vi "TestData_FileFormatCheck.vi"(8 "错误输入":errorcluster, 10 "Format Err":path, 11 "File":path) -> (0 "错误输出":errorcluster, 1 "Err_Count":i32, 3 "OK_Data":string[](array[string]))   [LabVIEW 2012, in "Lib_UEL.ATE.lvlib" / "Lib_TestData.lvlib"]
uses:
  Lib_TestData.lvlib
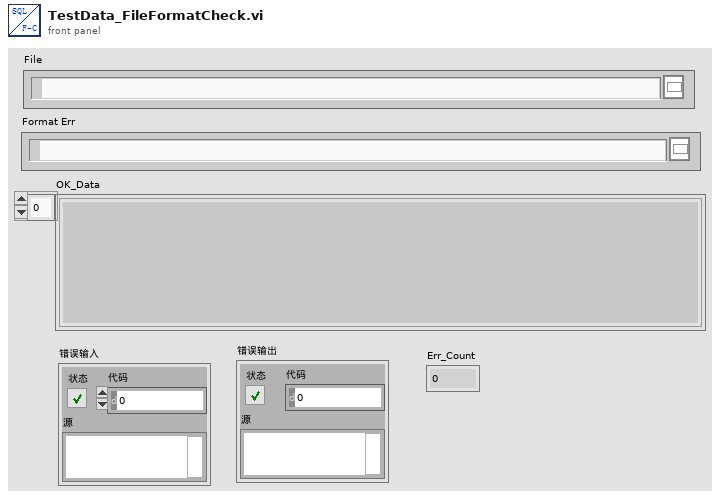
[diagram p1: front panel]
types:
  T1 = enum16{"open", "replace", "create", "open or create", "replace or create", "replace or create with confirmation"}
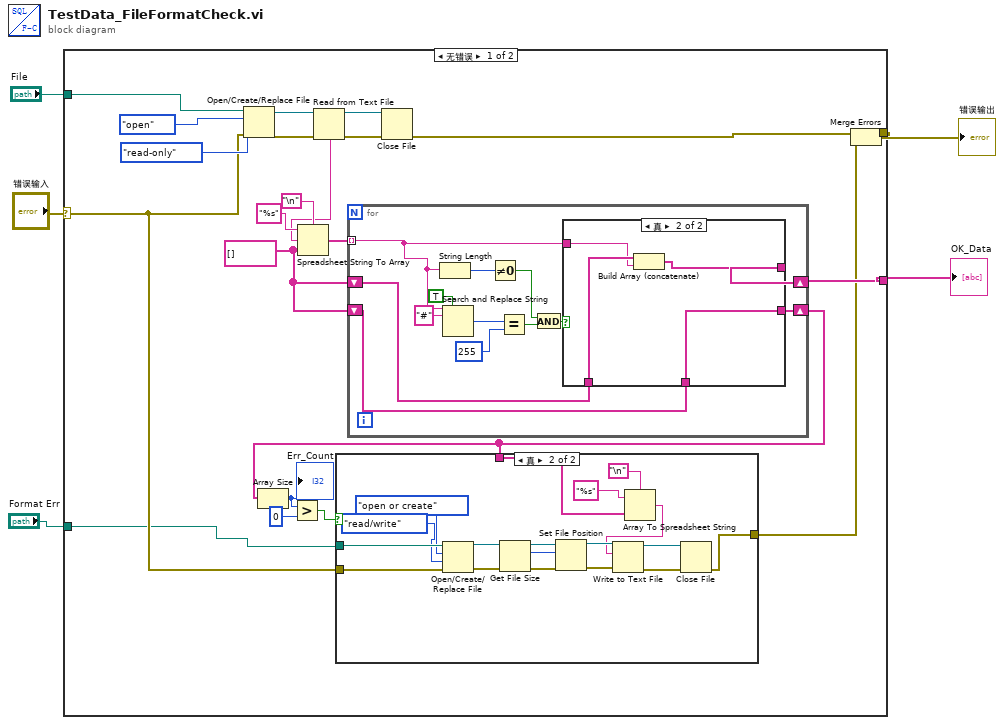
[diagram p0: block diagram]
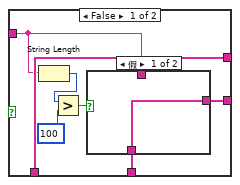
[diagram p3: hidden frame]
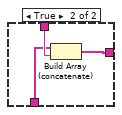
[diagram p4: hidden frame]
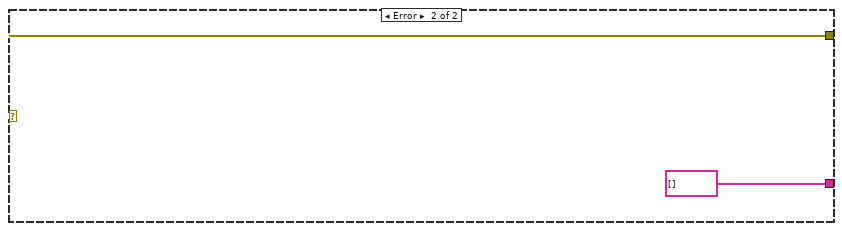
[diagram p5: hidden frame]
diagram:
  n1 = case shown="无错误" "错误输入" {
    selector: "错误输入" -> [w16 w76]
    tunnel: [w13 w76] -> w5
    tunnel: "File" -> [w18 _]
    tunnel: [w17 string[] []] -> w2
    tunnel: "Format Err" -> [w6 _]
    frame No Error {
      w7 = string[] []
      n2 = Open/Create/Replace File(file path (use dialog)=w18, error in=w16, operation (0:open)=T1."open" ("操作(0:open)"), access (0:read/write)=enum16{"read/write", "read-only", "write-only"}."read-only" ("权限(0:read/write)")) -> (refnum out=w27:refnum<file>, error out=w26:errorcluster)  [unwired: 2 in, 1 out]
      n3 = Read from Text File(file (use dialog)=w27, error in=w26) -> (refnum out=w25:refnum<file>, text=w19:string, error out=w24:errorcluster)  [unwired: 2 in, 1 out]
      n4 = Spreadsheet String To Array(delimiter (Tab)="\n", format string="%s" ("格式字符串"), spreadsheet string=w19, array type (2D Dbl)=w7) -> (array=w8:string[])
      n5 = for {
        tunnel: w8 -> [w49] mode=indexing
        shift-right: [w51] -> w17
        shift-left: w7 -> [w50]
        shift-right: [w48] -> w12
        shift-left: w7 -> [w47]
        n6 = String Length(string=w49) -> (length=w59:i32)
        n7 = Search and Replace String(replace all?=TRUE ("替换全部？(F)"), input string=w49, search string="#" ("搜索字符串")) -> (number of replacements=w56:i32)  [unwired: 5 in, 3 out]
        n8 = Not Equal To 0?(x=w59) -> (x != 0?=w53:bool)
        n9 = Equal?(x=w56, y=255) -> (x = y?=w54:bool)
        n10 = And(x=w53, y=w54) -> (x .and. y?=w52:bool)
        n11 = case shown="真" w52 {
          tunnel: w49 -> [w63 w72]
          tunnel: [w66 w74] -> w51
          tunnel: w50 -> [w66 w73]
          tunnel: [w65 w71] -> w48
          tunnel: w47 -> [w64 w71]
          frame False {
            n12 = String Length(string=w63) -> (length=w61:i32)
            n13 = Greater?(x=w61, y=100) -> (0:w62:bool)
            n14 = case shown="假" w62 {
              tunnel: w63 -> [_ w70]
              tunnel: [w67 w69] -> w65
              tunnel: w64 -> [w67 w68]
              frame False {
              }
              frame True {
                n15 = Build Array (concatenate)(w68, w70) -> (w69:string[])
              }
            }
          }
          frame True {
            n16 = Build Array (concatenate)(w73, w72) -> (w74:string[])
          }
        }
      }
      n17 = Array Size(array=w12) -> (size(s)=w11:i32)
      "Err_Count" <- w11
      n18 = Greater?(x=w11, y=0) -> (0:w9:bool)
      n19 = case shown="真" w9 {
        tunnel: w6 -> [_ w44]
        tunnel: w16 -> [w28 w43]
        tunnel: [w28 w38] -> w14
        tunnel: w12 -> [_ w37]
        frame False {
        }
        frame True {
          n20 = Open/Create/Replace File(file path (use dialog)=w44, error in=w43, operation (0:open)=T1."open or create" ("操作(0:open)"), access (0:read/write)=enum16{"read/write", "read-only", "write-only"}."read/write" ("权限(0:read/write)")) -> (refnum out=w36:refnum<file>, error out=w35:errorcluster)  [unwired: 2 in, 1 out]
          n21 = Get File Size(file=w36, error in=w35) -> (refnum out=w34:refnum<file>, size (in bytes)=w33:i64, 0:w32:errorcluster)
          n22 = Set File Position(offset (in bytes) (0)=w33, refnum=w34, error in=w32) -> (refnum out=w31:refnum<file>, error out=w30:errorcluster)  [unwired: 1 in]
          n23 = Array To Spreadsheet String(delimiter (Tab)="\n", array=w37, 3:"%s" ("格式字符串")) -> (spreadsheet string=w29:string)
          n24 = Write to Text File(file (use dialog)=w31, text=w29, error in=w30) -> (refnum out=w45:refnum<file>, error out=w46:errorcluster)  [unwired: 1 in, 1 out]
          n25 = Close File(refnum=w45, error in=w46) -> (error out=w38:errorcluster)  [unwired: 1 out]
        }
      }
      n26 = Close File(refnum=w25, error in=w24) -> (error out=w15:errorcluster)  [unwired: 1 out]
      n27 = Merge Errors(w15, w14) -> (w13:errorcluster)
    }
    frame Error {
    }
  }
  "错误输出" <- w5
  "OK_Data" <- w2
